vi "CThread Wait For Init.vi"   [LabVIEW 2012, in "CThread.lvlib"]
uses:
  CThread.lvlib
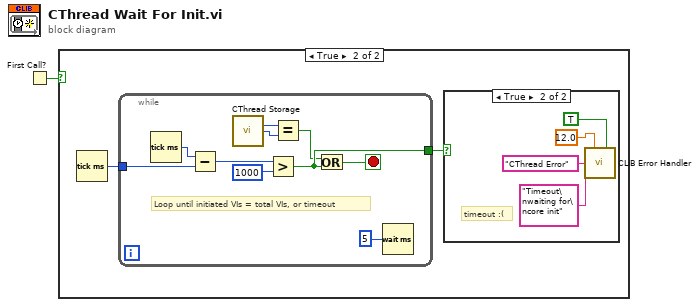
[diagram p0: block diagram]
diagram:
  n1 = First Call?() -> (First Call?: T/F=w1:bool)
  n2 = case shown="True" w1 {
    frame False {
    }
    frame True {
      n3 = Tick Count (ms)() -> (millisecond timer value=w3:u32)
      n4 = while {
        tunnel: w3 -> [w16]
        tunnel: [w15] -> w2
        stop <- w14 stop-if-true
        # "Loop until initiated VIs = total VIs, or timeout"
        n5 = Tick Count (ms)() -> (millisecond timer value=w17:u32)
        n6 = Subtract(x=w17, y=w16) -> (x-y=w10:u32)
        n7 = call "CThread Storage.vi"() -> ("# VIs Initiated"=w9:i32, "Total VIs"=w8:i32)  [unwired: 10 in, 4 out]
        n8 = Greater?(x=w10, y=1000) -> (0:w15:bool)
        n9 = Equal?(x=w9, y=w8) -> (x = y?=w13:bool)
        n10 = Or(x=w13, y=w15) -> (x .or. y?=w14:bool)
        n11 = Wait (ms)(milliseconds to wait=u32 5) -> ()  [unwired: 1 out]
      }
      n12 = case shown="True" w2 {
        frame False {
        }
        frame True {
          # "timeout :("
          n13 = call "CLIB Error Handler.vi"("Fatal Error? (T)"=TRUE, "Error Display Duration (5 sec)"=12.0, "Error Name"="CThread Error", "Error Description"="Timeout\nwaiting for\ncore init") -> ()  [unwired: 11 in, 1 out]
        }
      }
    }
  }
